vi "Restore Startup Configuration.vi"(8 "error in (no error)":errorcluster, 10 "Startup Configuration File":path=path "C:/Data/Config/start-up.cfg", 11 "Monitor-Pulse in":refnum<class "Application Controller.lvclass">) -> (0 "error out":errorcluster, 2 "Startup Configuration":T1={"Load Modules"=[], "External Modules Loaders"=[], "Root Data Folder"=path "C:/Data"}, 3 "Monitor-Pulse out":refnum<class "Application Controller.lvclass">)   [LabVIEW 2019, in "Application Controller.lvclass"]
uses:
  Application Controller.lvclass
  C:/GitHub/LabActor/Worker/Worker.lvclass
  Start-up Configuration.ctl
  Module Types.ctl
  Application Controller.lvclass/Application Controller.ctl
  Write Startup Configuration.vi
  <vilib>/Utility/error.llb/Error Cluster From Error Code.vi
  <vilib>/ErrorRing/Error Ring.xnode
  <vilib>/Utility/config.llb/NI_LVConfig.lvlib
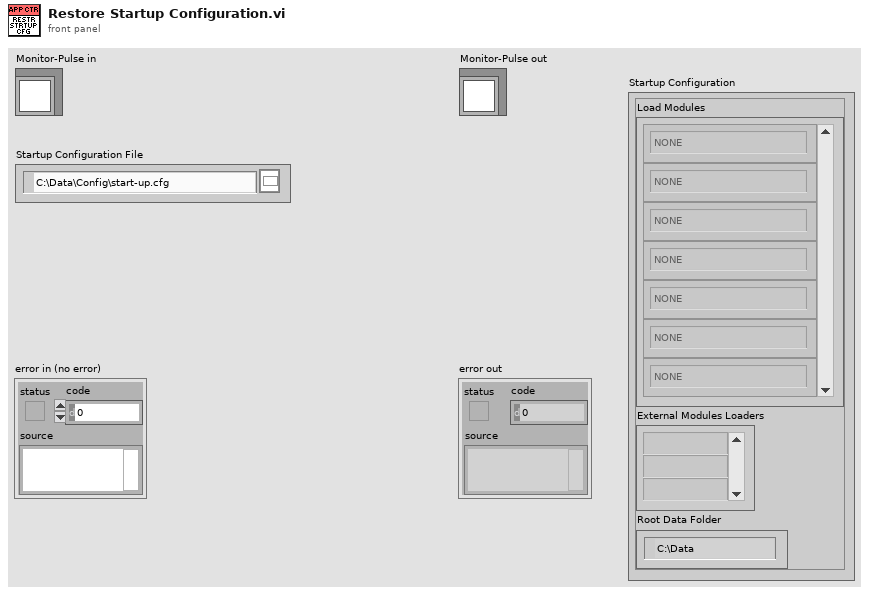
[diagram p1: front panel]
types:
  T1 = typedef "Start-up Configuration.ctl" = cluster{"Load Modules":T2[], "External Modules Loaders":string[], "Root Data Folder":path}
  T2 = typedef "Module Types.ctl" = enum16{"NONE", "NI-DAQmx", "NI-Scope", "Red Pitaya Digitizer", "GaGe", "VISA Device", "Red Pitaya Lockin", "Monitor Controller", "Pulse Controller", "Integrate Pulse", "Lockin Processor", "File converter", "NHMFL Synthesizer", "Micron Hyperion", "Spectrum Recorder", "Resonance Detector", "TCP Communications", "Format Resonances", "Ruby Spectra", "PID Controller", "Quantum Design", "VI Server"}
  T3 = typedef "NI_LVConfig.lvlib/Config Data RefNum.ctl" = refnum<k1>
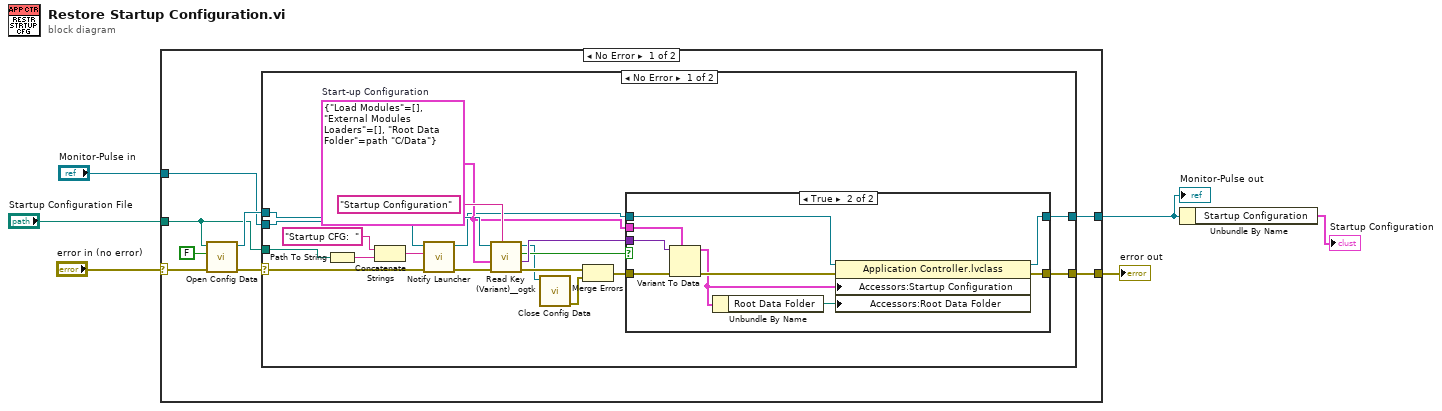
[diagram p0: block diagram]
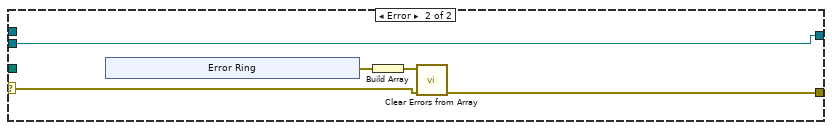
[diagram p3: hidden frame]
diagram:
  n1 = case shown="No Error" "error in (no error)" {
    selector: "error in (no error)" -> [w8 w55]
    tunnel: [w12 w55] -> w5
    tunnel: [w13 w54] -> w2
    tunnel: "Monitor-Pulse in" -> [w7 w54]
    tunnel: "Startup Configuration File" -> [w9 _]
    frame No Error {
      n2 = call <vilib>:"Open Config Data.vi"("error in (no error)"=w8, "create file if necessary (T)"=FALSE, "configuration file path"=w9) -> ("error out"=w11:errorcluster, "refnum"=w14:T3)  [unwired: 6 in, 1 out]
      n3 = case shown="No Error" w11 {
        selector: w11 -> [w22 w49]
        tunnel: w7 -> [w20 w48]
        tunnel: w14 -> [w32 _]
        tunnel: [w31 w48] -> w13
        tunnel: [w28 w47] -> w12
        tunnel: w9 -> [w18 _]
        frame No Error {
          w29 = T1 {"Load Modules"=[], "External Modules Loaders"=[], "Root Data Folder"=path "C:/Data"}  # Start-up Configuration
          n4 = Path To String(path=w18) -> (string=w16:string)
          n5 = Concatenate Strings("Startup CFG:  " ("notification"), w16) -> (w15:string)
          n6 = call-dynamic "Notify Launcher.vi"("error in (no error)"=w22, "Notification"=w15, "Application Controller in"=w20) -> ("error out"=w21:errorcluster, "Application Controller out"=w19:refnum<class "Application Controller.lvclass">)  [unwired: 7 in]
          n7 = call <userlib>:"Read Key (Variant)__ogtk.vi"("section"="Startup Configuration", "error in (no error)"=w21, "type"=w29, "refnum"=w32) -> ("error out"=w26:errorcluster, "key-value"=w30:variant, "found?"=w27:bool, "refnum out"=w25:T3)  [unwired: 4 in]
          n8 = call <vilib>:"Close Config Data.vi"("refnum"=w25) -> ("error out"=w24:errorcluster)  [unwired: 9 in, 1 out]
          n9 = Merge Errors(w26, w24) -> (w23:errorcluster)
          n10 = case shown="True" w27 {
            tunnel: w19 -> [w35 w39]
            tunnel: [w35 w38] -> w31
            tunnel: w23 -> [w34 w44]
            tunnel: w30 -> [_ w43]
            tunnel: w29 -> [_ w42]
            tunnel: [w34 w40] -> w28
            frame False {
            }
            frame True {
              n11 = Variant To Data(error in=w44, type=w42, Variant=w43) -> (data=w37:T1, error out=w41:errorcluster)
              n12 = Unbundle By Name(w37) -> ("Root Data Folder"=w36:path)
              n13 = property class="Application Controller.lvclass"(reference=w39, error in=w41, "Accessors:Startup Configuration"=w37, "Accessors:Root Data Folder"=w36) -> (reference out=w38:refnum<class "Application Controller.lvclass">, error out=w40:errorcluster)
            }
          }
        }
        frame Error {
          n14 = xnode "Error Ring"() -> ("error out"=w46:errorcluster)
          n15 = Build Array(w46) -> (w45:errorcluster[])
          n16 = call "Clear Errors from Array.vi"("Error In"=w49, "Errors to clear"=w45) -> ("Error Out"=w47:errorcluster)  [unwired: 8 in, 1 out]
        }
      }
    }
    frame Error {
    }
  }
  "error out" <- w5
  "Monitor-Pulse out" <- w2
  n17 = Unbundle By Name(w2) -> ("Startup Configuration"=→"Startup Configuration":T1)
